vi "Receive Message.vi"(6 "priority":i32, 10 "Actor in":refnum<class "Actor.lvclass">, 11 "Message in":refnum<class "Message.lvclass">) -> (0 "error out":errorcluster, 2 "Actor out":refnum<class "Actor.lvclass">)   [LabVIEW 2020, in "Actor Framework.lvlib" / "Actor.lvclass"]
doc: "This VI should be overriden ONLY if you are creating a proxy actor for remote transmission. If you are, override this VI to transmit the received message to a new destination, maintaining the given priority."
uses:
  Actor.lvclass
  Message/Message.lvclass
  Actor Framework.lvlib
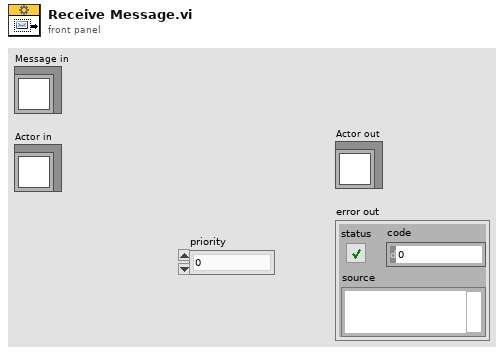
[diagram p1: front panel]
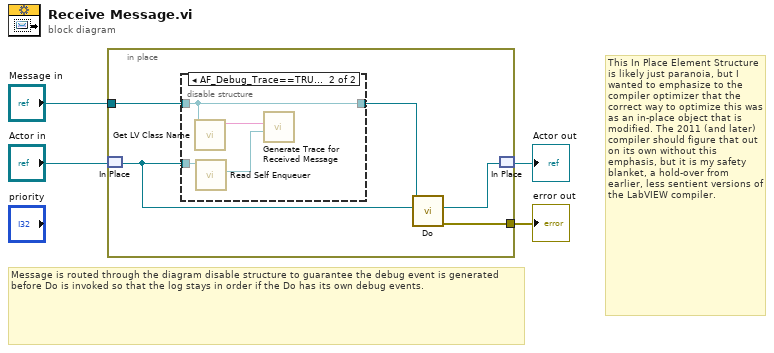
[diagram p0: block diagram]
diagram:
  # "Message is routed through the diagram disable structure to guarantee the debug event is generated before Do is invoked so that the log stays in order if the Do has its own debug events."
  # "This In Place Element Structure is likely just paranoia, but I wanted to emphasize to the compiler optimizer that the correct way to optimize this was as an in-place object that is modified. The 2011 (and later) compiler should figure that out on its own without this emphasis, but it is my safety blanket, a hold-over from earlier, less sentient versions of the LabVIEW compiler."
  n1 = in-place {
    in-place-border: [w9] -> w4
    in-place-border: "Message in" -> [w6]
    n2 = in-place-match #1("Actor in") -> (w7:refnum<class "Actor.lvclass">)
    n3 = disable-structure shown="AF_Debug_Trace==TRUE" {
      disable-tunnel: w7 -> [_ w14]
      disable-tunnel: w6 -> [w10 w13]
      disable-tunnel: [w10 w13] -> w5
      frame condition #0 (active) {
      }
      frame condition #1 {
        n4 = call <vilib>:"Get LV Class Name.vi"("object"=w13) -> ("class name"=w12:string)  [unwired: 9 in, 1 out]
        n5 = call "Read Self Enqueuer.vi"("Actor"=w14) -> ("Self Enqueuer"=w11:refnum<class "Message Enqueuer.lvclass">)  [unwired: 10 in]
        n6 = call "Generate Trace for Received Message.vi"("Actor"=w11, "Message Name"=w12) -> ()  [unwired: 10 in]
      }
    }
    n7 = call-dynamic "Do.vi"("Actor in"=w7, "Message"=w5) -> ("error out"=w9:errorcluster, "Actor out"=w8:refnum<class "Actor.lvclass">)  [unwired: 8 in]
    n8 = in-place-match #1(w8) -> (→"Actor out":refnum<class "Actor.lvclass">)
  }
  "error out" <- w4
